vi "RT Main.vi"   [LabVIEW 2021]
uses:
  <vilib>/FPGAPlugInAG/myRIO-1900/niLvFpga_Open_myRIO-1900.vi
  <vilib>/rvi/interface/common/dynamic/niFpgaDynamicAddResources.vi
  <vilib>/Utility/error.llb/Error Cluster From Error Code.vi
  <vilib>/rvi/errors/niLvFpgaAdjustHostInterfaceError.vi
  <vilib>/FPGAPlugInAG/Dynamic/niLvFpga_Close_Dynamic.vi
  <vilib>/rvi/interface/nirviOpenFPGA/nirviOpenFPGA.xnode
  FPGA Bitfiles/fpgaproject_FPGATarget_FPGAMain_zGCmK0Eh0KU.lvbitx
  FPGA Main.vi
  <vilib>/rvi/interface/nirviReadWriteControl/nirviReadWriteControl.xnode
  <vilib>/rvi/interface/nirviCloseFPGA/nirviCloseFPGA.xnode
  NiFpgaLv.dll
  <vilib>/rvi/interface/Simulation/niFpgaSimulationCallBeginRW.vi
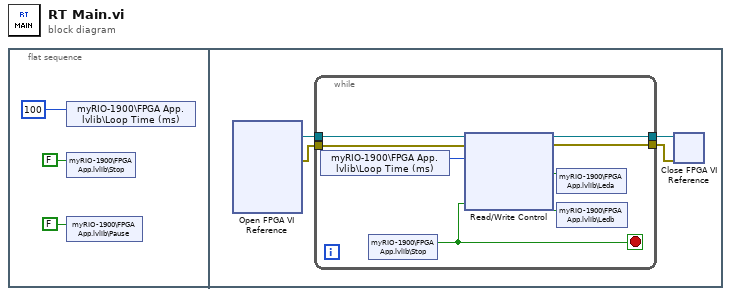
[diagram p0: block diagram]
diagram:
  n1 = flat-sequence {
    frame #0 {
      n2 = shared-variable "myRIO-1900\\FPGA App.lvlib\\Loop Time (ms)"(u32 100 ("Loop Time (ms)")) -> ()  [unwired: 1 in, 1 out]
      n3 = shared-variable "myRIO-1900\\FPGA App.lvlib\\Stop"(FALSE ("Paused")) -> ()  [unwired: 1 in, 1 out]
      n4 = shared-variable "myRIO-1900\\FPGA App.lvlib\\Pause"(FALSE ("Pause")) -> ()  [unwired: 1 in, 1 out]
    }
    frame #1 {
      n5 = xnode "Open FPGA VI Reference"() -> ("FPGA VI Reference Out"=w7:refnum<k20>, "error out"=w6:errorcluster)  [unwired: 2 in]
      n6 = while {
        tunnel: w7 -> [w15]
        tunnel: w6 -> [w14]
        tunnel: [w10] -> w5
        tunnel: [w9] -> w4
        stop <- w8 stop-if-true
        n7 = shared-variable "myRIO-1900\\FPGA App.lvlib\\Loop Time (ms)"() -> (w13:u32)  [unwired: 1 in, 1 out]
        n8 = shared-variable "myRIO-1900\\FPGA App.lvlib\\Stop"() -> (w8:bool)  [unwired: 1 in, 1 out]
        n9 = xnode "Read/Write Control"("FPGA VI Reference In"=w15, "error in"=w14, "Count(mSec)"=w13, "Pause"=w8) -> ("FPGA VI Reference Out"=w10:refnum<k20>, "error out"=w9:errorcluster, "Led0i"=w12:bool, "Led1i"=w11:bool)
        n10 = shared-variable "myRIO-1900\\FPGA App.lvlib\\Leda"(w12) -> ()  [unwired: 1 in, 1 out]
        n11 = shared-variable "myRIO-1900\\FPGA App.lvlib\\Ledb"(w11) -> ()  [unwired: 1 in, 1 out]
      }
      n12 = xnode "Close FPGA VI Reference"("FPGA VI Reference In"=w5, "error in"=w4) -> ()  [unwired: 1 out]
    }
  }
